vi "Test_DDS_to_host.vi"() -> ()   [LabVIEW 2013]
uses:
  <vilib>/userdefined/High Color/nirio_resource_hc.ctl
  <vilib>/FPGAPlugInAG/PXIe-7975R/niLvFpga_Open_PXIe-7975R.vi
  <vilib>/rvi/interface/common/dynamic/niFpgaDynamicAddResources.vi
  <vilib>/rvi/interface/common/niFpgaWaitOnOcc.vi
  <vilib>/Utility/error.llb/Error Cluster From Error Code.vi
  <vilib>/rvi/errors/niLvFpgaAdjustHostInterfaceError.vi
  <vilib>/rvi/interface/nirviOpenFPGA/nirviOpenFPGA.xnode
  FPGA Bitfiles/FPGAoutputfromDDS_to_host_T1B3HnZlK8A.lvbitx
  <vilib>/rvi/interface/nirviMethod/nirviMethod.xnode
  <vilib>/rvi/interface/nirviReadWriteControl/nirviReadWriteControl.xnode
  <vilib>/rvi/errors/niLvFpgaMergeErrorWithErrorCode.vi
  <vilib>/FPGAPlugInAG/Dynamic/niLvFpga_ReadFifo_Dynamic.vi
  <vilib>/FPGAPlugInAG/Dynamic/niLvFpga_ConfigureFifo_Dynamic.vi
  <vilib>/FPGAPlugInAG/Dynamic/niLvFpga_StartFifo_Dynamic.vi
  NiFpgaLv.dll
  <vilib>/rvi/interface/Simulation/niFpgaSimulationCallBeginRW.vi
panel:
  in  "stop":bool
  out "Elements Remaining":u32
  out "error out":errorcluster
  out "size(s)":i32
  out "Data":u64[](array[numeric])
  in  "Output mixer fequency [MHz]":dbl
  in  "Run":bool
  in  "#samples":u16
  out "Actual Depth":u32
  in  "resource name":T1="RIO0"
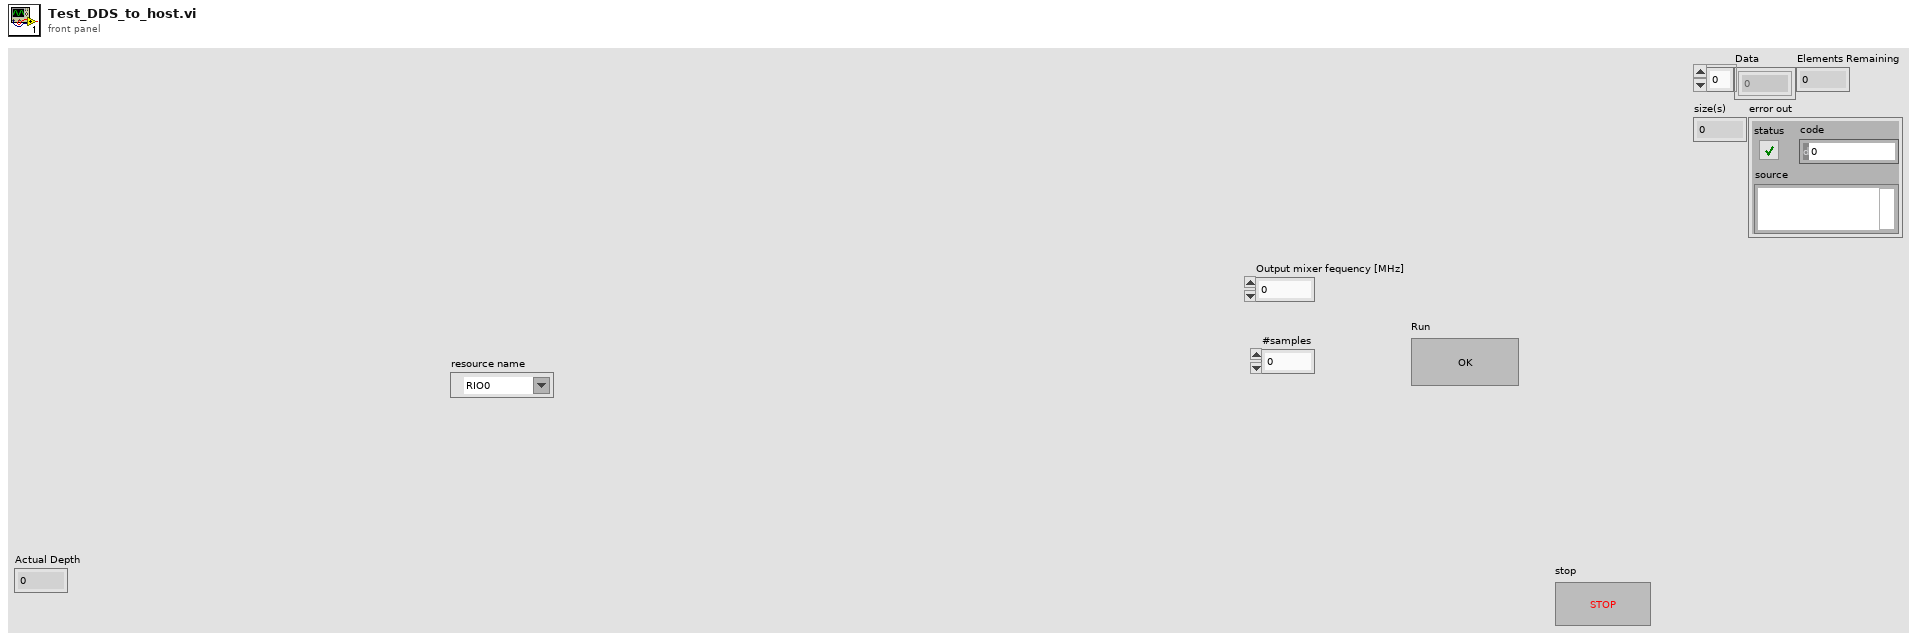
[diagram p1: front panel]
types:
  T1 = typedef "nirio_resource_hc.ctl" = tag
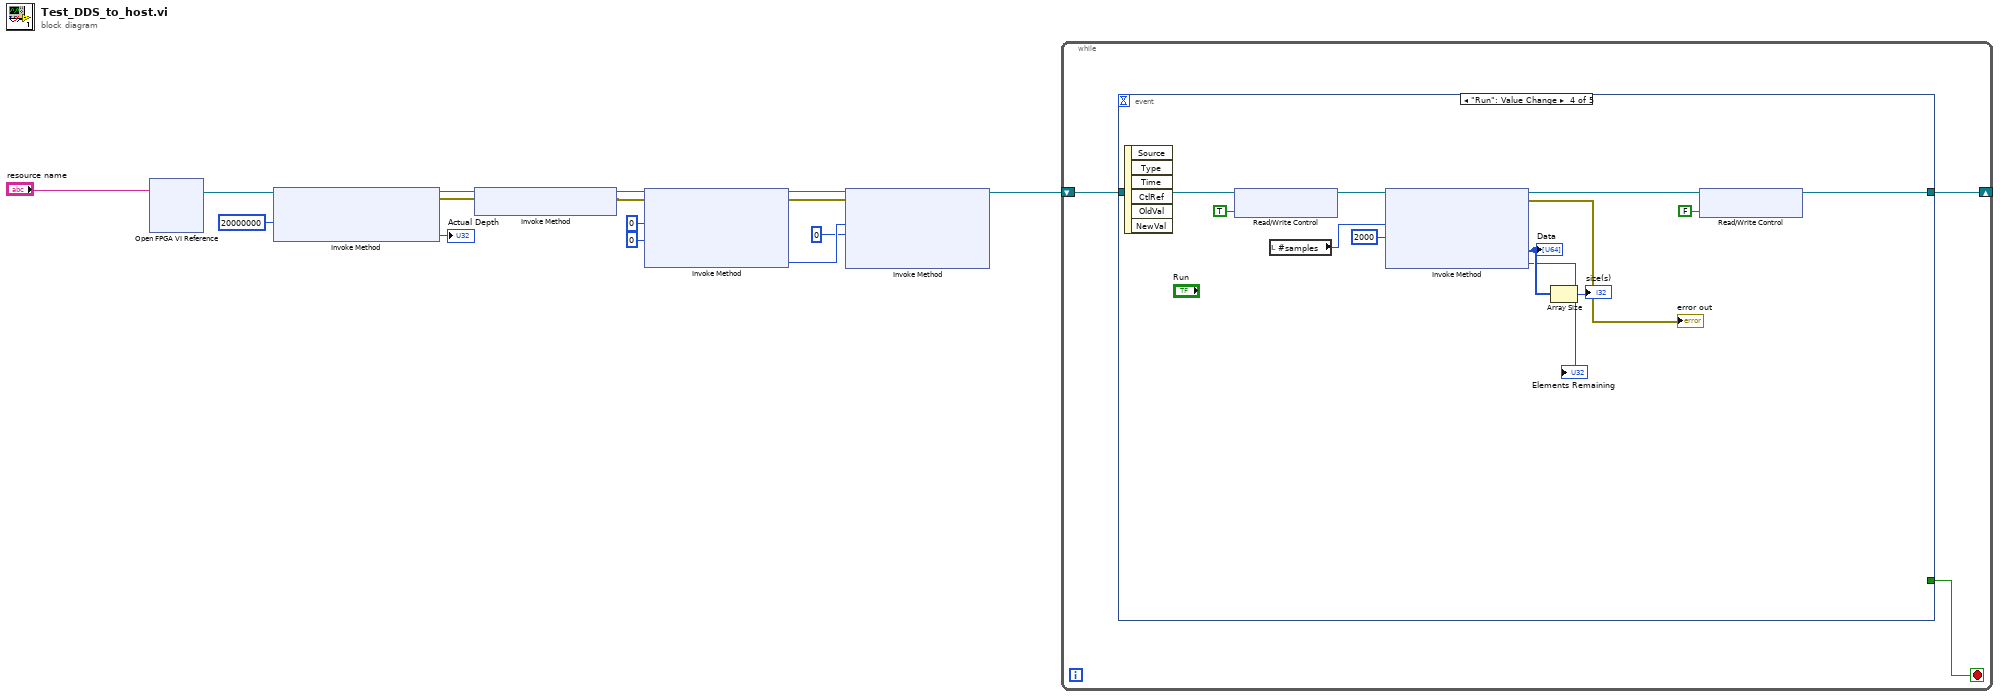
[diagram p0: block diagram]
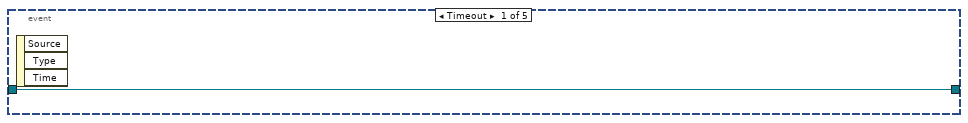
[diagram p2: hidden frame]
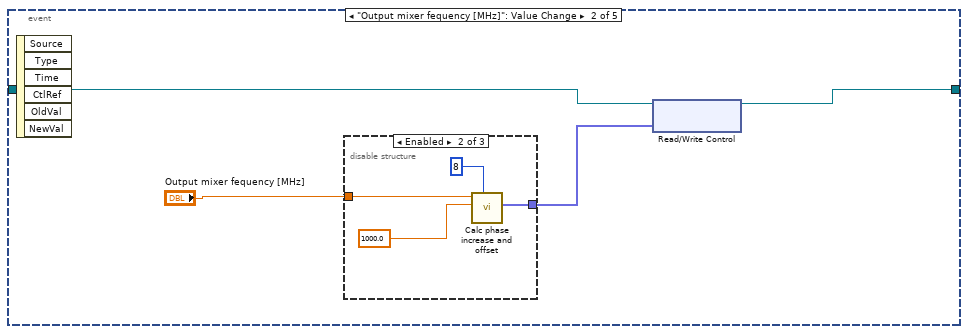
[diagram p3: hidden frame]
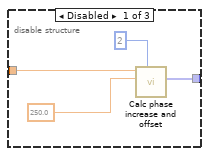
[diagram p4: hidden frame]
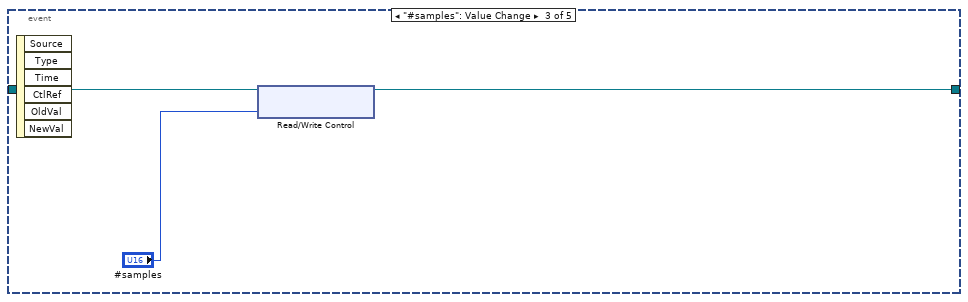
[diagram p6: hidden frame]
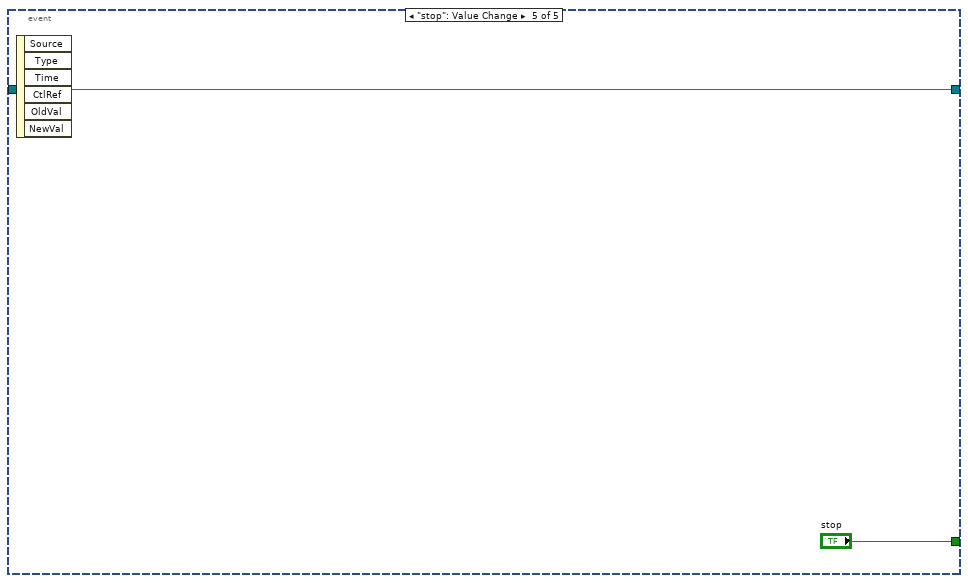
[diagram p7: hidden frame]
diagram:
  n1 = xnode "Open FPGA VI Reference"("resource name"="resource name") -> ("FPGA VI Reference Out"=w2:refnum<k20>)  [unwired: 1 in, 1 out]
  n2 = xnode "Invoke Method"("FPGA VI Reference In"=w2, "Requested Depth"=u32 20000000 ("Depth")) -> ("FPGA VI Reference Out"=w12:refnum<k20>, "error out"=w13:errorcluster, "Actual Depth"=→"Actual Depth":u32)  [unwired: 1 in]
  n3 = xnode "Invoke Method"("FPGA VI Reference In"=w12, "error in"=w13) -> ("FPGA VI Reference Out"=w4:refnum<k20>, "error out"=w3:errorcluster)
  n4 = xnode "Invoke Method"("FPGA VI Reference In"=w4, "error in"=w3, "Number of Elements"=u32 0, "Timeout (ms)"=0) -> ("FPGA VI Reference Out"=w7:refnum<k20>, "error out"=w6:errorcluster, "Elements Remaining"=w9:u32)  [unwired: 1 out]
  n5 = xnode "Invoke Method"("FPGA VI Reference In"=w7, "error in"=w6, "Number of Elements"=w9, "Timeout (ms)"=0) -> ("FPGA VI Reference Out"=w1:refnum<k20>)  [unwired: 3 out]
  n6 = while {
    shift-right: [w18] -> _
    shift-left: w1 -> [w17]
    stop <- w16 stop-if-true
    n7 = event shown="[3] \"Run\": Value Change" {
      selector: _ -> [_ _ _ _ _]
      dyn-events: _ -> [_ _ _ _ _]
      timeout: _ -> [_ _ _ _ _]
      tunnel: [w19 w21 w32 w36 w48] -> w18
      tunnel: w17 -> [w19 w20 w34 w46 w48]
      tunnel: [_ _ _ _ "stop"] -> w16
      event Timeout {
        n8 = event-data() -> ()  [unwired: 1 in, 3 out]
      }
      event "Output mixer fequency [MHz]": Value Change {
        n9 = event-data() -> ()  [unwired: 1 in, 6 out]
        n10 = disable-structure shown="Enabled" {
          disable-tunnel: [w25 w29 _] -> w22
          disable-tunnel: "Output mixer fequency [MHz]" -> [w24 w28 _]
          frame Disabled {
            n11 = call "Calc phase increase and offset.vi"("# of DDS"=2, "fclk (MHz)"=250.0 ("fclk (800MHz)"), "f_generated (MHz)"=w24) -> ("Phase out"=w25:fxp<+,64,64>[])  [unwired: 6 in, 2 out]
          }
          frame Enabled {
            n12 = call "Calc phase increase and offset.vi"("# of DDS"=8, "fclk (MHz)"=1000.0 ("fclk (800MHz)"), "f_generated (MHz)"=w28) -> ("Phase out"=w29:fxp<+,64,64>[])  [unwired: 6 in, 2 out]
          }
          frame Disabled {
          }
        }
        n13 = xnode "Read/Write Control"("FPGA VI Reference In"=w20, "Phase output"=w22) -> ("FPGA VI Reference Out"=w21:refnum<k20>)  [unwired: 1 in, 1 out]
      }
      event "#samples": Value Change {
        n14 = event-data() -> ()  [unwired: 1 in, 6 out]
        n15 = xnode "Read/Write Control"("FPGA VI Reference In"=w34, "5782 record length"="#samples") -> ("FPGA VI Reference Out"=w32:refnum<k20>)  [unwired: 1 in, 1 out]
      }
      event "Run": Value Change {
        n16 = event-data() -> ()  [unwired: 1 in, 6 out]
        n17 = xnode "Read/Write Control"("FPGA VI Reference In"=w46, "Trigger Acquisition"=TRUE) -> ("FPGA VI Reference Out"=w44:refnum<k20>)  [unwired: 1 in, 1 out]
        n18 = local read "#samples"() -> (w43:u16)
        n19 = xnode "Invoke Method"("FPGA VI Reference In"=w44, "Number of Elements"=w43, "Timeout (ms)"=2000) -> ("FPGA VI Reference Out"=w37:refnum<k20>, "error out"=→"error out":errorcluster, "Data"=w41:u64[], "Elements Remaining"=→"Elements Remaining":u32)  [unwired: 1 in]
        "Data" <- w41
        n20 = Array Size(array=w41) -> (size(s)=→"size(s)":i32)
        n21 = xnode "Read/Write Control"("FPGA VI Reference In"=w37, "Trigger Acquisition"=FALSE) -> ("FPGA VI Reference Out"=w36:refnum<k20>)  [unwired: 1 in, 1 out]
      }
      event "stop": Value Change {
        n22 = event-data() -> ()  [unwired: 1 in, 6 out]
      }
    }
  }
